vi "LvMPDC_SUB_TCPRead.vi"(8 "error in (no error)":errorcluster, 9 "timeout_ms":i32=1000, 10 "ReadBytes":i32=10240, 11 "Connect ID":refnum<k5>) -> (0 "error out":errorcluster, 2 "Recv String":string, 3 "Connect ID out":refnum<k5>)   [LabVIEW 2012]
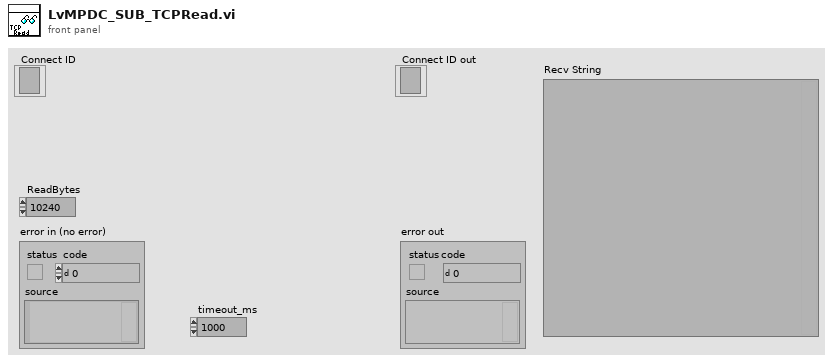
[diagram p1: front panel]
types:
  T1 = enum16{"Standard", "Buffered", "CRLF", "Immediate"}
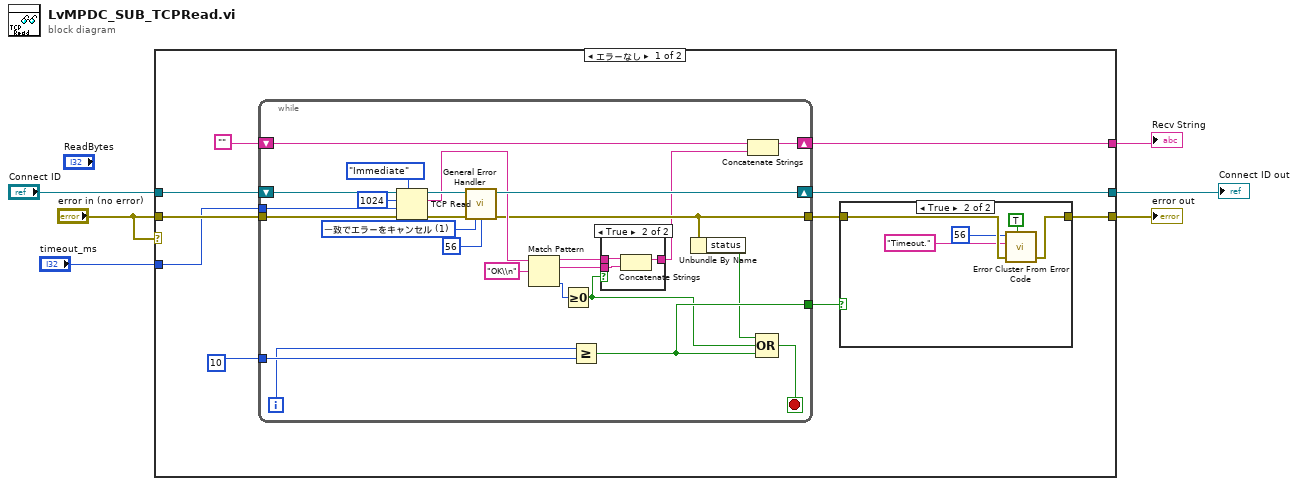
[diagram p0: block diagram]
diagram:
  n1 = case shown="エラーなし" "error in (no error)" {
    tunnel: "Connect ID" -> [w16 w52]
    tunnel: [w15 w52] -> w5
    tunnel: [w13 _] -> w4
    tunnel: "error in (no error)" -> [w12 w51]
    tunnel: [w7 w51] -> w3
    tunnel: "timeout_ms" -> [w11 _]
    frame No Error {
      n2 = while {
        shift-right: [w41] -> w13
        shift-left: "" -> [w42]
        shift-right: [w43] -> w15
        shift-left: w16 -> [w44]
        tunnel: w12 -> [w40]
        tunnel: [w28] -> w8
        tunnel: w11 -> [w36]
        tunnel: 10 -> [w31]
        tunnel: [w29] -> w9
        i -> [w30]
        stop <- w32 stop-if-true
        w39 = 1 items=["例外なし", "一致でエラーをキャンセル", "一致でエラーをセット"] ("[exception action] (none:0)")
        n3 = TCP Read(connection ID=w44, bytes to read=1024 ("読み取りバイト数"), error in (no error)=w40, 7:T1."Immediate" ("モード（標準）"), 9:w36) -> (connection ID out=w43:refnum<k5>, data out=w33:string, error out=w37:errorcluster)
        n4 = call <vilib>:"General Error Handler.vi"("error in (no error)"=w37, "[exception action] (none:0)"=w39, "[exception code]"=56) -> ("error out"=w28:errorcluster)  [unwired: 8 in, 4 out]
        n5 = Match Pattern(string=w33, regular expression="OK\\n" ("正規表現")) -> (before substring=w25:string, match substring=w24:string, offset past match=w34:i32)  [unwired: 1 in, 1 out]
        n6 = Greater Or Equal To 0?(x=w34) -> (x >= 0?=w26:bool)
        n7 = Greater Or Equal?(x=w30, y=w31) -> (x >= y?=w29:bool)
        n8 = case shown="TRUE" w26 {
          tunnel: w25 -> [w47 w50]
          tunnel: w24 -> [_ w49]
          tunnel: [w47 w48] -> w23
          frame False {
          }
          frame True {
            n9 = Concatenate Strings(w50, w49) -> (w48:string)
          }
        }
        n10 = Unbundle By Name(w28) -> ("status"=w27:bool)
        n11 = Concatenate Strings(w42, w23) -> (w41:string)
        n12 = Compound Arithmetic op=OR(w27, w26, w29) -> (w32:bool)
      }
      n13 = case shown="TRUE" w9 {
        tunnel: w8 -> [w17 w22]
        tunnel: [w17 w21] -> w7
        frame False {
        }
        frame True {
          n14 = call <vilib>:"Error Cluster From Error Code.vi"("show call chain? (False)"=TRUE, "error in (no error)"=w22, "error message (\"\")"="Timeout." ("error message (\"\")"), "error code (0)"=56) -> ("error out"=w21:errorcluster)  [unwired: 5 in]
        }
      }
    }
    frame Error {
    }
  }
  "Connect ID out" <- w5
  "error out" <- w3
  "Recv String" <- w4
